vi "Init.vi"(8 "error in (no error)":errorcluster, 11 "QuickSilver in":refnum<class "QuickSilver.lvclass">) -> (0 "error out":errorcluster, 3 "QuickSilver out":refnum<class "QuickSilver.lvclass">)   [LabVIEW 2018, in "QuickSilver.lvclass"]
uses:
  QuickSilver.lvclass
  QuickSilver.lvclass/QuickSilver.ctl
  <vilib>/Instr/_visa.llb/VISA Configure Serial Port (Instr).vi
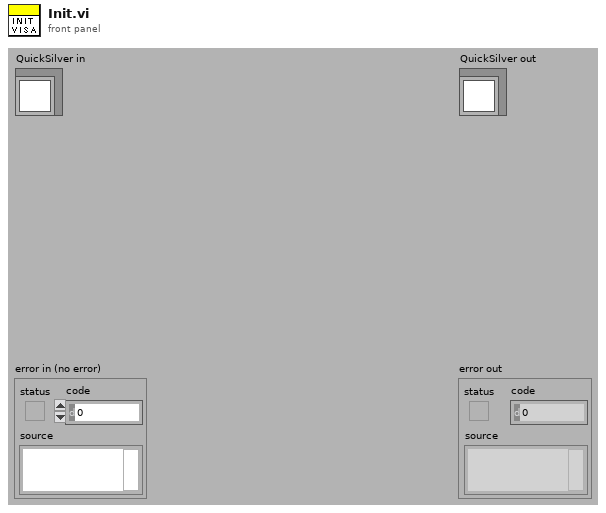
[diagram p1: front panel]
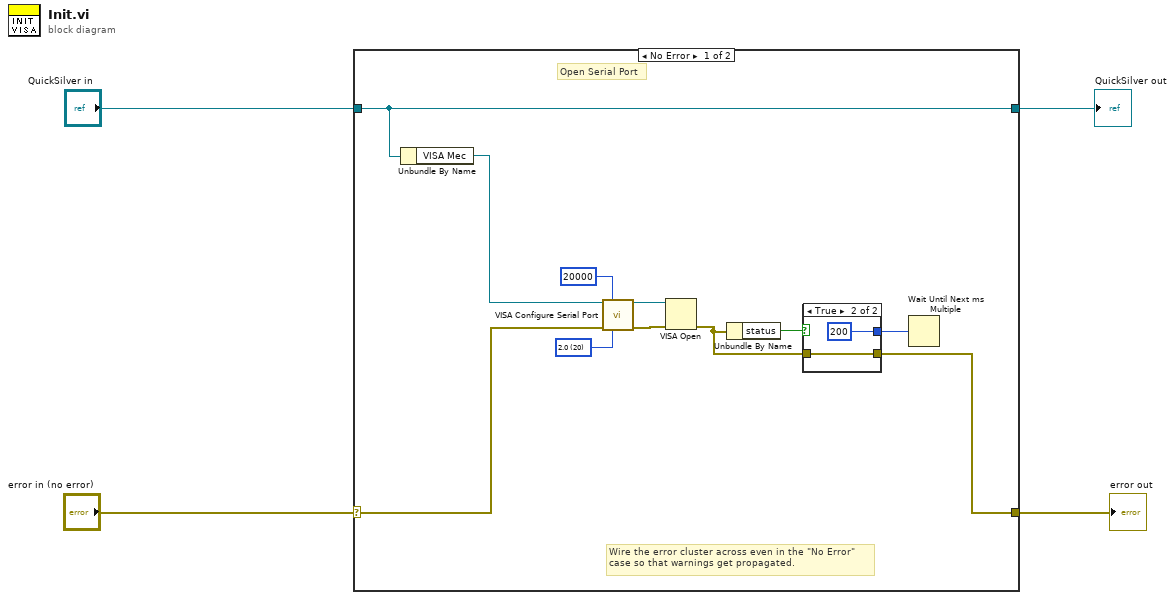
[diagram p0: block diagram]
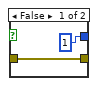
[diagram p2: hidden frame]
diagram:
  n1 = case shown="No Error" "error in (no error)" {
    selector: "error in (no error)" -> [w9 w21]
    tunnel: [w14 w21] -> w2
    tunnel: [w15 w20] -> w1
    tunnel: "QuickSilver in" -> [w15 w20]
    frame No Error {
      w8 = u16 20 items=["1.0"=10, "1.5"=15, "2.0"=20] ("stop bits (10: 1 bit)")
      # "Wire the error cluster across even in the \"No Error\"\ncase so that warnings get propagated."
      # "Open Serial Port"
      n2 = Unbundle By Name(w15) -> ("VISA Mec"=w10:refnum<visa-resource-name>)
      n3 = call-poly "VISA Configure Serial Port"("VISA resource name"=w10, "timeout (10sec)"=u32 20000, "error in (no error)"=w9, "stop bits (10: 1 bit)"=w8) -> ("VISA resource name out"=w6:refnum<visa-resource-name>, "error out"=w5:errorcluster)  [unwired: 4 in, 6 out]
      n4 = VISA Open(error in (no error)=w5, VISA resource name=w6) -> (error out=w11:errorcluster)  [unwired: 4 out]
      n5 = Unbundle By Name(w11) -> ("status"=w12:bool)
      n6 = case shown="True" w12 {
        tunnel: [1 200] -> w13
        tunnel: w11 -> [w17 w18]
        tunnel: [w17 w18] -> w14
        frame False {
        }
        frame True {
        }
      }
      n7 = Wait Until Next ms Multiple(millisecond multiple=w13) -> ()  [unwired: 1 out]
    }
    frame Error {
    }
  }
  "error out" <- w2
  "QuickSilver out" <- w1
